vi "AlignDelayStage.vi"() -> ()   [LabVIEW 2017]
uses:
  Newport ESP301/Newport ESP301.lvlib
panel:
  out "Moving":bool
  out "Scanning":bool
  in  "home":bool
  out "Current Position (mm)":sgl=72.92 format="%.3f"
  out "At 2":bool
  out "At 1":bool
  in  "(Wait per mm (s/mm))":dbl=0.038
  out "Added Wait (s)":dbl
  in  "Go 2":bool
  in  "Go 1":bool
  in  "Position 2 (mm)":dbl=-90.0
  in  "start":bool
  in  "Position 1 (mm)":dbl=90.0
  in  "= Wait 1?":bool
  in  "Wait 2 (s)":dbl=10.0
  in  "Wait 1 (s)":dbl=10.0
  in  "stop":bool
  out "error out":errorcluster {"code" format="%.0x"}
  in  "error in (no error)":errorcluster
  in  "ESP301 Serial":string="1"
  in  "Axis":i32=2 min=1 max=3 step=1
  out "ESP301 VISA Session":string
  # "Controller for Delay Stage Alignment"
  # "Stage\nMoving"
  # "Stage Controller Properties"
  # "All movement LED indicators \nbased on calculated wait time!"
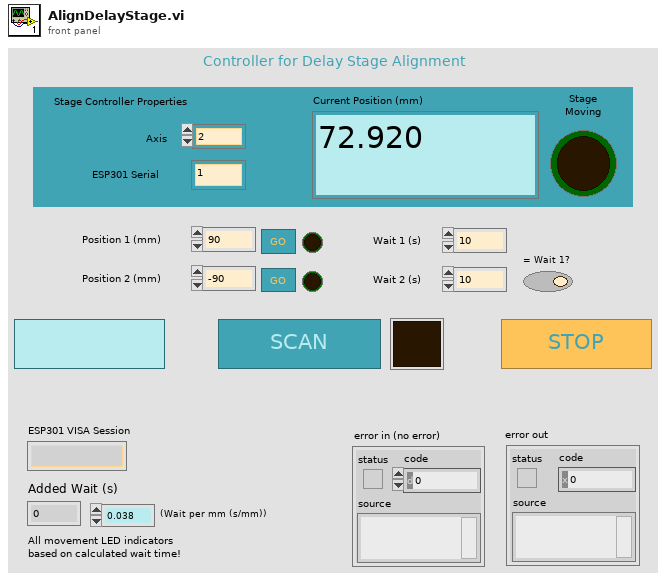
[diagram p1: front panel]
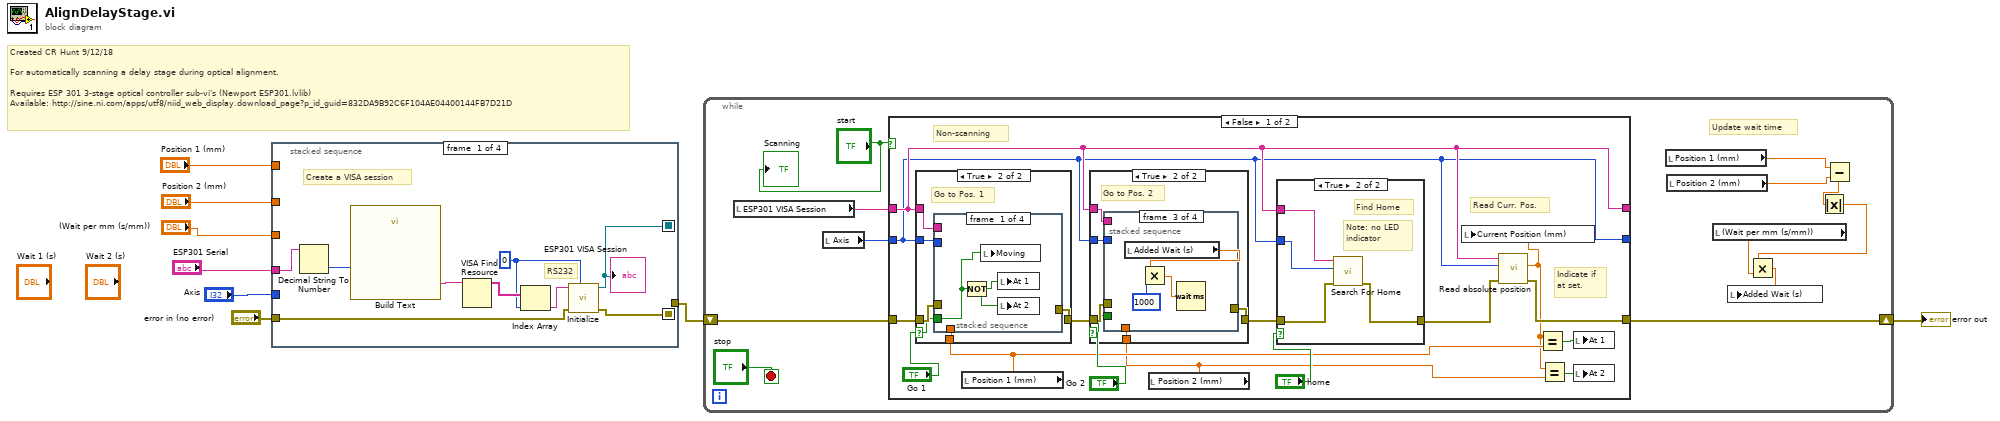
[diagram p0: block diagram]
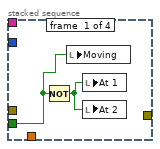
[diagram p4: hidden frame]
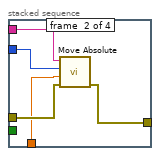
[diagram p5: hidden frame]
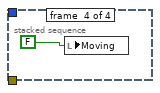
[diagram p6: hidden frame]
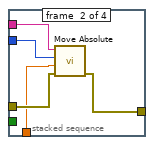
[diagram p8: hidden frame]
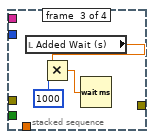
[diagram p9: hidden frame]
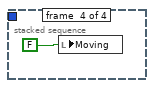
[diagram p10: hidden frame]
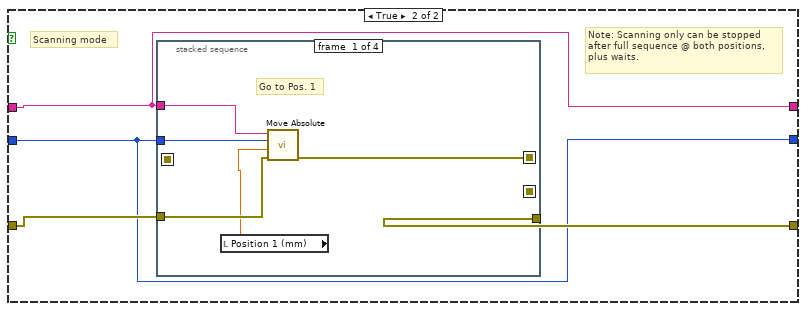
[diagram p11: hidden frame]
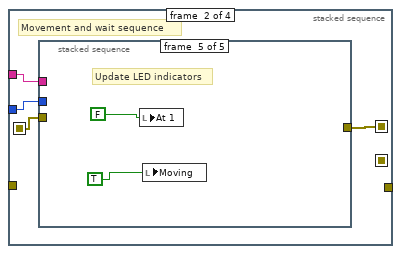
[diagram p12: hidden frame]
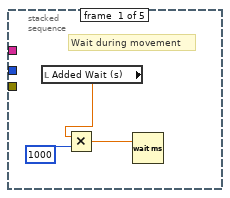
[diagram p13: hidden frame]
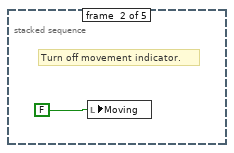
[diagram p14: hidden frame]
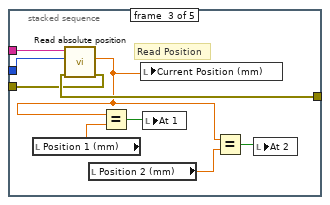
[diagram p15: hidden frame]
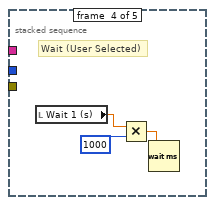
[diagram p16: hidden frame]
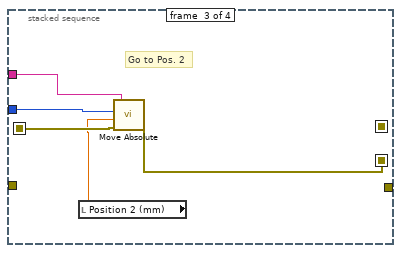
[diagram p17: hidden frame]
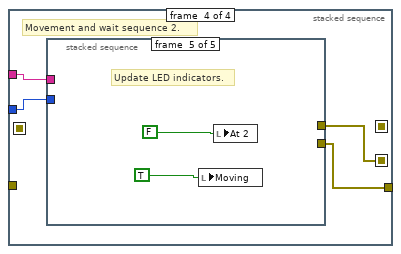
[diagram p18: hidden frame]
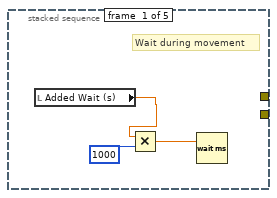
[diagram p19: hidden frame]
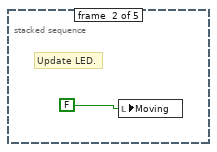
[diagram p20: hidden frame]
diagram:
  # "Created CR Hunt 9/12/18\n\nFor automatically scanning a delay stage during optical alignment.\n\nRequires ESP 301 3-stage optical controller sub-vi's (Newport ESP301.lvlib)\nAvailable: http://sine.ni.com/apps/utf8/niid_web_display.download_page?p_id_guid=832DA9B92C6F104AE04400144FB7D21D"
  n1 = stacked-sequence {
    seq-local: [w10 _ _ _] -> [_ _ w26 _]
    seq-local: [w9 _ _ _] -> [_ _ w25 _]
    tunnel: "ESP301 Serial" -> [w17 _ _ _]
    tunnel: "error in (no error)" -> [w11 _ _ _]
    tunnel: "Position 1 (mm)" -> [_ w21 w28 _]
    tunnel: "Position 2 (mm)" -> [_ w20 w27 _]
    tunnel: "Axis" -> [_ _ w30 _]
    tunnel: [_ _ w29 _] -> w2
    tunnel: "(Wait per mm (s/mm))" -> [_ w19 _ _]
    frame #0 {
      w13 = 0
      # "RS232"
      # "Create a VISA session"
      n2 = Decimal String To Number(string=w17) -> (number=w16:i32)  [unwired: 2 in, 1 out]
      n3 = call "Build Text"("port_number"=w16) -> ("Result"=w15:string)  [unwired: 13 in, 1 out]
      n4 = VISA Find Resource(11:w15) -> (3:w14:string[])  [unwired: 2 in, 2 out]
      n5 = Index Array(array=w14, index=w13) -> (element=w12:string)
      n6 = call "Initialize.vi"("VISA resource name"=w12, "error in (no error)"=w11, "Serial Link (RS232)"=w13) -> ("VISA resource name out"=w9:refnum<visa-resource-name>, "error out"=w10:errorcluster)  [unwired: 6 in]
      "ESP301 VISA Session" <- w9
    }
    frame #1 {
      w18 = FALSE
      # "Initialize LEDs"
      # "Calculate wait time for motor\nmovement"
      n7 = Subtract(x=w21, y=w20) -> (x-y=w24:dbl)
      n8 = Absolute Value(x=w24) -> (abs(x)=w23:dbl)
      n9 = Multiply(x=w23, y=w19) -> (x*y=→"Added Wait (s)":dbl)
      "At 2" <- w18
      "At 1" <- w18
      "Moving" <- w18
    }
    frame #2 {
      # "Indicate if\nat setpoint"
      # "Read current position"
      n10 = call "Read absolute position.vi"("error in (no error)"=w26, "Axis (1)"=w30, "VISA resource name"=w25) -> ("error out"=w29:errorcluster, "Position (units)"=w31:dbl)  [unwired: 2 in, 1 out]
      "Current Position (mm)" <- w31
      n11 = Equal?(x=w28, y=w31) -> (x = y?=w33:bool)
      n12 = Equal?(x=w27, y=w31) -> (x = y?=w32:bool)
      n13 = local write "At 1"(w33) -> ()
      n14 = local write "At 2"(w32) -> ()
    }
    frame #3 {
      # "Deep breath"
      n15 = Wait (ms)(milliseconds to wait=200) -> ()  [unwired: 1 out]
    }
  }
  n16 = while {
    shift-right: [w36] -> w6
    shift-left: w2 -> [w45]
    stop <- "stop" stop-if-true
    # "Update wait time"
    n17 = local read "ESP301 VISA Session"() -> (w44:string)
    n18 = local read "Axis"() -> (w43:i32)
    n19 = case shown="False" "start" {
      tunnel: w45 -> [w61 w106]
      tunnel: [w52 w105] -> w36
      tunnel: w44 -> [w55 w104]
      tunnel: w43 -> [w54 w103]
      tunnel: [w55 w104] -> _
      tunnel: [w54 w103] -> _
      frame False {
        # "Non-scanning"
        # "Indicate if\nat set."
        # "Read Curr. Pos."
        n20 = local read "Position 1 (mm)"() -> (w51:dbl)
        n21 = case shown="True" "Go 1" {
          selector: "Go 1" -> [_ w87]
          tunnel: w61 -> [w85 w88]
          tunnel: [w85 w86] -> w60
          tunnel: w55 -> [_ w91]
          tunnel: w54 -> [_ w90]
          tunnel: w51 -> [_ w89]
          frame False {
          }
          frame True {
            # "Go to Pos. 1"
            n22 = stacked-sequence {
              tunnel: w88 -> [_ w98 _ _]
              tunnel: [_ w97 _ _] -> w86
              tunnel: w91 -> [_ w96 _ _]
              tunnel: w90 -> [_ w95 _ _]
              tunnel: w89 -> [_ w94 _ _]
              tunnel: w87 -> [w92 _ _ _]
              frame #0 {
                n23 = Not(x=w92) -> (.not. x?=w93:bool)
                n24 = local write "Moving"(w92) -> ()
                n25 = local write "At 1"(w93) -> ()
                n26 = local write "At 2"(w93) -> ()
              }
              frame #1 {
                n27 = call "Move Absolute.vi"("error in (no error)"=w98, "Position (0 units)"=w94, "Axis (1)"=w95, "VISA resource name"=w96) -> ("error out"=w97:errorcluster)  [unwired: 2 in, 1 out]
              }
              frame #2 {
                n28 = local read "Added Wait (s)"() -> (w99:dbl)
                n29 = Multiply(x=w99, y=1000) -> (x*y=w100:dbl)
                n30 = Wait (ms)(milliseconds to wait=w100) -> ()  [unwired: 1 out]
              }
              frame #3 {
                n31 = local write "Moving"(FALSE) -> ()
              }
            }
          }
        }
        n32 = local read "Position 2 (mm)"() -> (w50:dbl)
        n33 = case shown="True" "Go 2" {
          selector: "Go 2" -> [_ w70]
          tunnel: w60 -> [w67 w71]
          tunnel: [w67 w68] -> w57
          tunnel: w55 -> [_ w73]
          tunnel: w54 -> [_ w72]
          tunnel: w50 -> [_ w69]
          frame False {
          }
          frame True {
            # "Go to Pos. 2"
            n34 = stacked-sequence {
              tunnel: w71 -> [_ w80 _ _]
              tunnel: [_ w79 _ _] -> w68
              tunnel: w73 -> [_ w78 _ _]
              tunnel: w72 -> [_ w77 _ _]
              tunnel: w69 -> [_ w76 _ _]
              tunnel: w70 -> [w74 _ _ _]
              frame #0 {
                n35 = Not(x=w74) -> (.not. x?=w75:bool)
                n36 = local write "Moving"(w74) -> ()
                n37 = local write "At 1"(w75) -> ()
                n38 = local write "At 2"(w75) -> ()
              }
              frame #1 {
                n39 = call "Move Absolute.vi"("error in (no error)"=w80, "Position (0 units)"=w76, "Axis (1)"=w77, "VISA resource name"=w78) -> ("error out"=w79:errorcluster)  [unwired: 2 in, 1 out]
              }
              frame #2 {
                n40 = local read "Added Wait (s)"() -> (w81:dbl)
                n41 = Multiply(x=w81, y=1000) -> (x*y=w82:dbl)
                n42 = Wait (ms)(milliseconds to wait=w82) -> ()  [unwired: 1 out]
              }
              frame #3 {
                n43 = local write "Moving"(FALSE) -> ()
              }
            }
          }
        }
        n44 = case shown="True" "home" {
          tunnel: w57 -> [w62 w66]
          tunnel: [w62 w65] -> w53
          tunnel: w55 -> [_ w64]
          tunnel: w54 -> [_ w63]
          frame False {
          }
          frame True {
            # "Note: no LED\nindicator"
            # "Find Home"
            n45 = call "Search For Home.vi"("error in (no error)"=w66, "Axis (1)"=w63, "VISA resource name"=w64) -> ("error out"=w65:errorcluster)  [unwired: 4 in, 1 out]
          }
        }
        n46 = call "Read absolute position.vi"("error in (no error)"=w53, "Axis (1)"=w54, "VISA resource name"=w55) -> ("error out"=w52:errorcluster, "Position (units)"=w47:dbl)  [unwired: 2 in, 1 out]
        n47 = local write "Current Position (mm)"(w47) -> ()
        n48 = Equal?(x=w47, y=w51) -> (x = y?=w49:bool)
        n49 = Equal?(x=w47, y=w50) -> (x = y?=w48:bool)
        n50 = local write "At 1"(w49) -> ()
        n51 = local write "At 2"(w48) -> ()
      }
      frame True {
        # "Note: Scanning only can be stopped\nafter full sequence @ both positions,\nplus waits."
        # "Scanning mode"
        n52 = stacked-sequence {
          seq-local: [w110 _ _ _] -> [_ w115 _ _]
          seq-local: [_ w114 _ _] -> [_ _ w138 _]
          seq-local: [_ _ w137 _] -> [_ _ _ w142]
          tunnel: w106 -> [w111 _ _ _]
          tunnel: [_ _ _ w141] -> w105
          tunnel: w104 -> [w109 w113 w136 w140]
          tunnel: w103 -> [w108 w112 w135 w139]
          frame #0 {
            # "Go to Pos. 1"
            n53 = local read "Position 1 (mm)"() -> (w107:dbl)
            n54 = call "Move Absolute.vi"("error in (no error)"=w111, "Position (0 units)"=w107, "Axis (1)"=w108, "VISA resource name"=w109) -> ("error out"=w110:errorcluster)  [unwired: 2 in, 1 out]
          }
          frame #1 {
            # "Movement and wait sequence"
            n55 = stacked-sequence {
              tunnel: w115 -> [_ _ w128 _ _]
              tunnel: [_ _ w127 _ _] -> w114
              tunnel: w113 -> [_ _ w126 _ _]
              tunnel: w112 -> [_ _ w125 _ _]
              frame #0 {
                # "Wait during movement"
                n56 = local read "Added Wait (s)"() -> (w116:dbl)
                n57 = Multiply(x=w116, y=1000) -> (x*y=w118:dbl)
                n58 = Wait (ms)(milliseconds to wait=w118) -> ()  [unwired: 1 out]
              }
              frame #1 {
                # "Turn off movement indicator."
                n59 = local write "Moving"(FALSE) -> ()
              }
              frame #2 {
                # "Read Position"
                n60 = local read "Position 1 (mm)"() -> (w124:dbl)
                n61 = call "Read absolute position.vi"("error in (no error)"=w128, "Axis (1)"=w125, "VISA resource name"=w126) -> ("error out"=w127:errorcluster, "Position (units)"=w121:dbl)  [unwired: 2 in, 1 out]
                n62 = local read "Position 2 (mm)"() -> (w122:dbl)
                n63 = Equal?(x=w121, y=w124) -> (x = y?=w123:bool)
                n64 = local write "Current Position (mm)"(w121) -> ()
                n65 = local write "At 1"(w123) -> ()
                n66 = Equal?(x=w121, y=w122) -> (x = y?=w120:bool)
                n67 = local write "At 2"(w120) -> ()
              }
              frame #3 {
                # "Wait (User Selected)"
                n68 = local read "Wait 1 (s)"() -> (w131:dbl)
                n69 = Multiply(x=w131, y=1000) -> (x*y=w129:dbl)
                n70 = Wait (ms)(milliseconds to wait=w129) -> ()  [unwired: 1 out]
              }
              frame #4 {
                # "Update LED indicators"
                n71 = local write "At 1"(FALSE) -> ()
                n72 = local write "Moving"(TRUE) -> ()
              }
            }
          }
          frame #2 {
            # "Go to Pos. 2"
            n73 = local read "Position 2 (mm)"() -> (w134:dbl)
            n74 = call "Move Absolute.vi"("error in (no error)"=w138, "Position (0 units)"=w134, "Axis (1)"=w135, "VISA resource name"=w136) -> ("error out"=w137:errorcluster)  [unwired: 2 in, 1 out]
          }
          frame #3 {
            # "Movement and wait sequence 2."
            n75 = stacked-sequence {
              tunnel: w142 -> [_ _ w155 _ _]
              tunnel: w140 -> [_ _ w154 _ _]
              tunnel: w139 -> [_ _ w153 _ _]
              tunnel: [_ _ w150 _ _] -> w141
              frame #0 {
                # "Wait during movement"
                n76 = local read "Added Wait (s)"() -> (w143:dbl)
                n77 = Multiply(x=w143, y=1000) -> (x*y=w145:dbl)
                n78 = Wait (ms)(milliseconds to wait=w145) -> ()  [unwired: 1 out]
              }
              frame #1 {
                # "Update LED."
                n79 = local write "Moving"(FALSE) -> ()
              }
              frame #2 {
                # "Read Pos."
                n80 = local read "Position 2 (mm)"() -> (w151:dbl)
                n81 = local read "Position 1 (mm)"() -> (w148:dbl)
                n82 = call "Read absolute position.vi"("error in (no error)"=w155, "Axis (1)"=w153, "VISA resource name"=w154) -> ("error out"=w150:errorcluster, "Position (units)"=w147:dbl)  [unwired: 2 in, 1 out]
                n83 = local write "Current Position (mm)"(w147) -> ()
                n84 = Equal?(x=w147, y=w151) -> (x = y?=w152:bool)
                n85 = Equal?(x=w147, y=w148) -> (x = y?=w149:bool)
                n86 = local write "At 2"(w152) -> ()
                n87 = local write "At 1"(w149) -> ()
              }
              frame #3 {
                # "Wait (User Selected)"
                n88 = case shown="True" "= Wait 1?" {
                  tunnel: [w160 w161] -> w156
                  frame False {
                    n89 = local read "Wait 2 (s)"() -> (w160:dbl)
                  }
                  frame True {
                    n90 = local read "Wait 1 (s)"() -> (w161:dbl)
                    n91 = local write "Wait 2 (s)"(w161) -> ()
                  }
                }
                n92 = Multiply(x=w156, y=1000) -> (x*y=w158:dbl)
                n93 = Wait (ms)(milliseconds to wait=w158) -> ()  [unwired: 1 out]
              }
              frame #4 {
                # "Update LED indicators."
                n94 = local write "Moving"(TRUE) -> ()
                n95 = local write "At 2"(FALSE) -> ()
              }
            }
          }
        }
      }
    }
    n96 = local read "Position 1 (mm)"() -> (w38:dbl)
    n97 = local read "Position 2 (mm)"() -> (w37:dbl)
    n98 = local read "(Wait per mm (s/mm))"() -> (w39:dbl)
    n99 = Subtract(x=w38, y=w37) -> (x-y=w41:dbl)
    n100 = Absolute Value(x=w41) -> (abs(x)=w42:dbl)
    n101 = Multiply(x=w42, y=w39) -> (x*y=w40:dbl)
    n102 = local write "Added Wait (s)"(w40) -> ()
    "Scanning" <- "start"
  }
  "error out" <- w6
